vi "TDMS Read.vi"() -> ()   [LabVIEW 2017]
panel:
  out "found":bool
  out "property value":string
  out "Waveform Chart":waveform(dbl)[](graph)
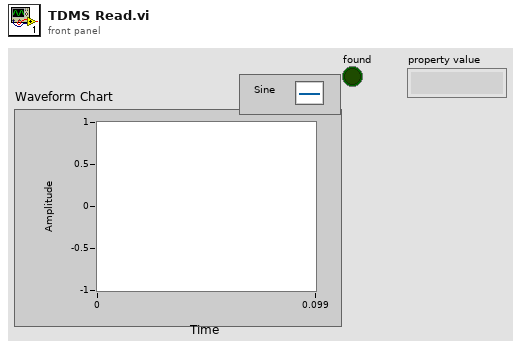
[diagram p1: front panel]
types:
  T1 = enum16{"open", "open or create", "create or replace", "create", "open (read-only)"}
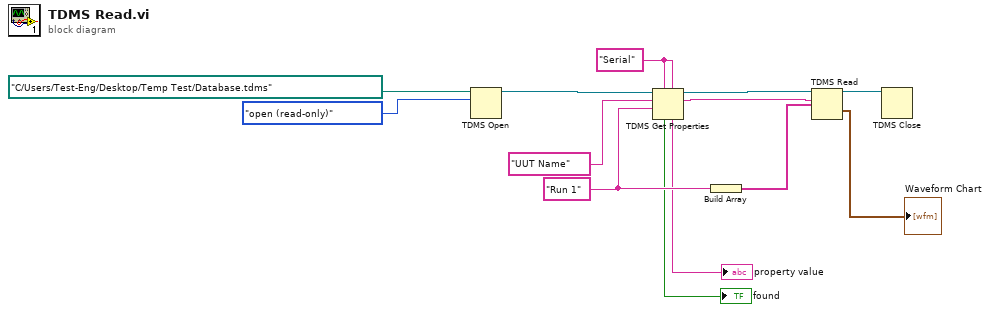
[diagram p0: block diagram]
diagram:
  w1 = "Serial" ("property name")
  w7 = "Run 1" ("channel name")
  n1 = TDMS Open(10:T1."open (read-only)" ("operation (0:open)"), 11:path "C:/Users/Test-Eng/Desktop/Temp Test/Database.tdms" ("file path")) -> (3:w11:refnum<k34>)  [unwired: 5 in, 1 out]
  n2 = TDMS Get Properties(5:w1, 7:w1, 9:w7, 10:"UUT Name" ("group name in (Untitled)"), 11:w11) -> (2:w5:string, 3:w10:refnum<k34>, 4:→"property value":string, 6:→"found":bool)  [unwired: 1 in, 2 out]
  n3 = Build Array(w7) -> (w6:string[])
  n4 = TDMS Read(0:w10, 5:w5, 7:w6) -> (4:w8:refnum<k34>, 10:→"Waveform Chart":waveform(dbl)[])  [unwired: 5 in, 4 out]
  n5 = TDMS Close(11:w8) -> ()  [unwired: 1 in, 2 out]
